vi "Arduino Wait for Move Complete.vi"(8 "error in (no error)":errorcluster, 11 "reference":refnum<visa-resource-name>) -> (0 "error out":errorcluster, 1 "response":string, 2 "distance":i32, 3 "Motor":i32)   [LabVIEW 2021, in "FW Arduino Control.lvclass"]
uses:
  FW Arduino Control.lvclass
  ef667a97-bf22-4261-9fe2-826bdb4b0545.vi
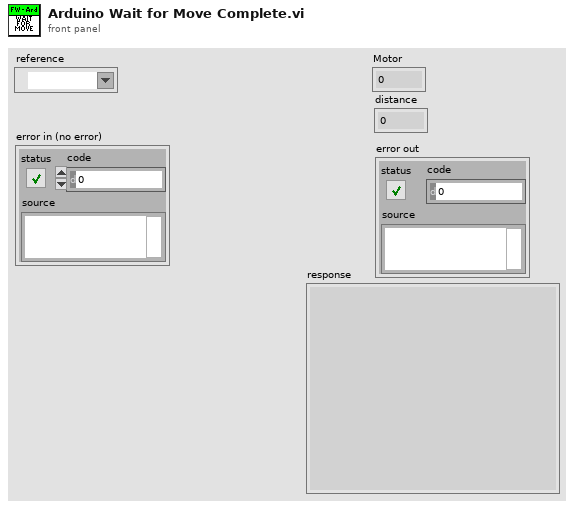
[diagram p1: front panel]
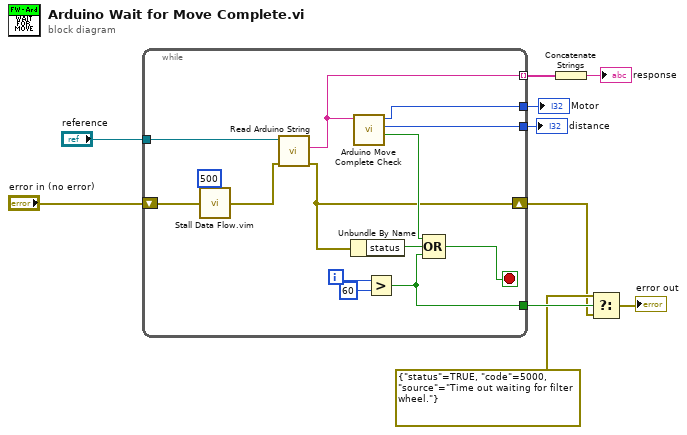
[diagram p0: block diagram]
diagram:
  n1 = while {
    tunnel: "reference" -> [w24]
    shift-right: [w13] -> w4
    shift-left: "error in (no error)" -> [w23]
    tunnel: [w18] -> w8
    tunnel: [w17] -> w7
    tunnel: [w12] -> w6
    tunnel: [w11] -> w2 mode=indexing
    i -> [w15]
    stop <- w16 stop-if-true
    n2 = call "Stall Data Flow.vim"("value in"=w23, "milliseconds to wait"=u32 500) -> ("value out"=w21:errorcluster)  [unwired: 1 out]
    n3 = call "Read Arduino String.vi"("error in (no error)"=w21, "reference"=w24) -> ("error out"=w13:errorcluster, "response"=w11:string)  [unwired: 7 in, 1 out]
    n4 = Unbundle By Name(w13) -> ("status"=w20:bool)
    n5 = call "Arduino Move Complete Check.vi"("input string"=w11) -> ("Complete?"=w19:bool, "position"=w17:i32, "m"=w18:i32)  [unwired: 8 in]
    n6 = Greater?(x=w15, y=60) -> (0:w12:bool)
    n7 = Compound Arithmetic op=OR(w19, w20, w12) -> (w16:bool)
  }
  "Motor" <- w8
  "distance" <- w7
  n8 = Concatenate Strings(w2) -> (→"response":string)
  n9 = Select(t=errorcluster {"status"=TRUE, "code"=5000, "source"="Time out waiting for filter wheel."} ("error in (no error)"), s=w6, f=w4) -> (s? t:f=→"error out":errorcluster)
